vi "get_settings_cluster.vi"(8 "error in (no error)":errorcluster, 11 "GenericPlugin in":refnum<class "DetectorDL090603DAQmxOnOff.lvclass">) -> (0 "error out":errorcluster, 2 "settings cluster":variant, 3 "GenericPlugin out":refnum<class "DetectorDL090603DAQmxOnOff.lvclass">)   [LabVIEW 2011, in "DetectorDL090603DAQmxOnOff.lvclass"]
uses:
  DetectorDL090603DAQmxOnOff.lvclass
  DetectorDL090603DAQmxOnOff.lvclass/DetectorDL090603DAQmxOnOff.ctl
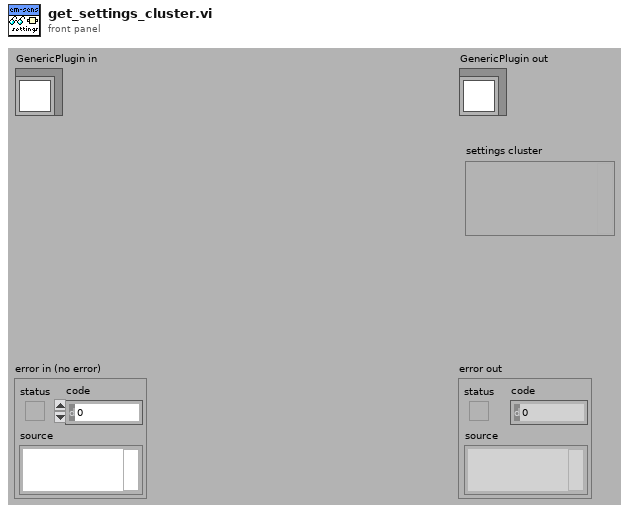
[diagram p1: front panel]
types:
  T1 = typedef "DetectorDL090603DAQmxOnOff.lvclass/settings_cluster.ctl" = cluster{"voltage":dbl[unit]}
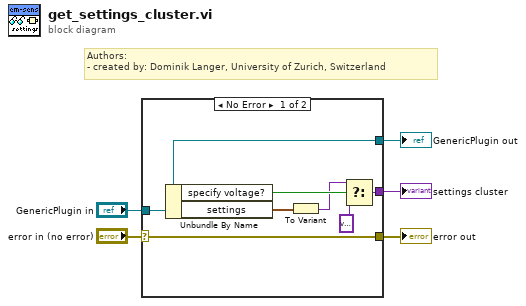
[diagram p0: block diagram]
diagram:
  # "Authors: \n- created by: Dominik Langer, University of Zurich, Switzerland"
  n1 = case shown="No Error" "error in (no error)" {
    selector: "error in (no error)" -> [w11 w13]
    tunnel: "GenericPlugin in" -> [w10 w14]
    tunnel: [w7 _] -> w4
    tunnel: [w11 w13] -> w2
    tunnel: [w10 w14] -> w1
    frame No Error {
      n2 = Unbundle By Name(w10) -> ("specify voltage?"=w9:bool, "settings"=w12:T1)
      n3 = To Variant(anything=w12) -> (Variant=w8:variant)
      n4 = Select(t=w8, s=w9, f=variant) -> (s? t:f=w7:variant)
    }
    frame Error {
    }
  }
  "error out" <- w2
  "GenericPlugin out" <- w1
  "settings cluster" <- w4
